vi "Offline_Analysis_SWSVM_newSelectionMethod_in_분석기.vi"(0 "LDA_matrix":path caption="LDA_matrix.txt", 1 "Target":path, 2 "Nontarget":path, 3 "in_matrix":path caption="in", 5 "svm_model_file":string, 7 "Target_order.txt":path, 9 "mius_flash_order":path, 11 "Brain":path, 12 "피험자이름":string="홍길동", 13 "Save_path":string) -> ()   [LabVIEW 2013]
uses:
  <vilib>/Utility/file.llb/Read From Spreadsheet File (DBL).vi
  <vilib>/Utility/file.llb/Read From Spreadsheet File (I64).vi
  <vilib>/Utility/file.llb/Write To Spreadsheet File (DBL).vi
  <vilib>/Utility/file.llb/Write To Spreadsheet File (I64).vi
  <vilib>/Utility/file.llb/Write To Spreadsheet File (string).vi
  <vilib>/Analysis/Matrix/NI_Matrix.lvlib
  <vilib>/Analysis/Matrix/Numeric/Conversions/Array To Matrix - RA2.vi
  <vilib>/Analysis/Matrix/Numeric/Conversions/Array To Matrix - RA.vi
panel:
  out "ACC":i16
  out "Target_order":i64[](array[numeric])
  out "Selected_Target":i32[](array[numeric])
  out "Accuracy":i16[](array[numeric])
  out "error out":errorcluster
  in  "Random_num":i32=6
  in  "Flash_Repeat":i32=20
  in  "Frame_Length":i32=10
  in  "Sampling_Rate":dbl=250.0
  # "ERP_Parameter안씀. LDA바로 집어넣으면 됨"
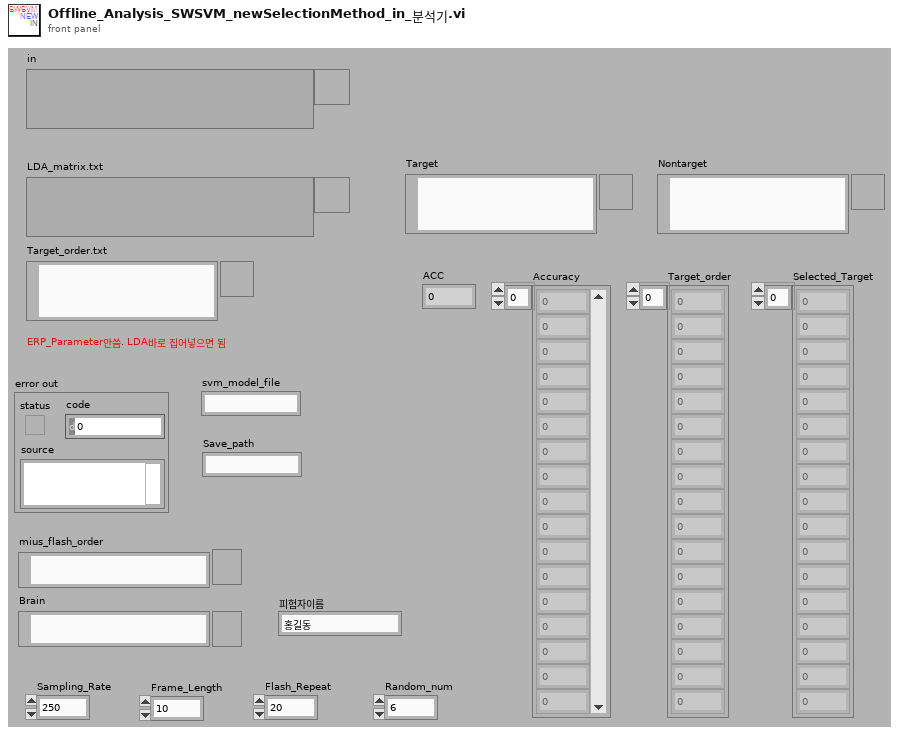
[diagram p1: front panel]
types:
  T1 = typedef "NI_Matrix.lvlib/RealMatrix.ctl" = dbl[][]
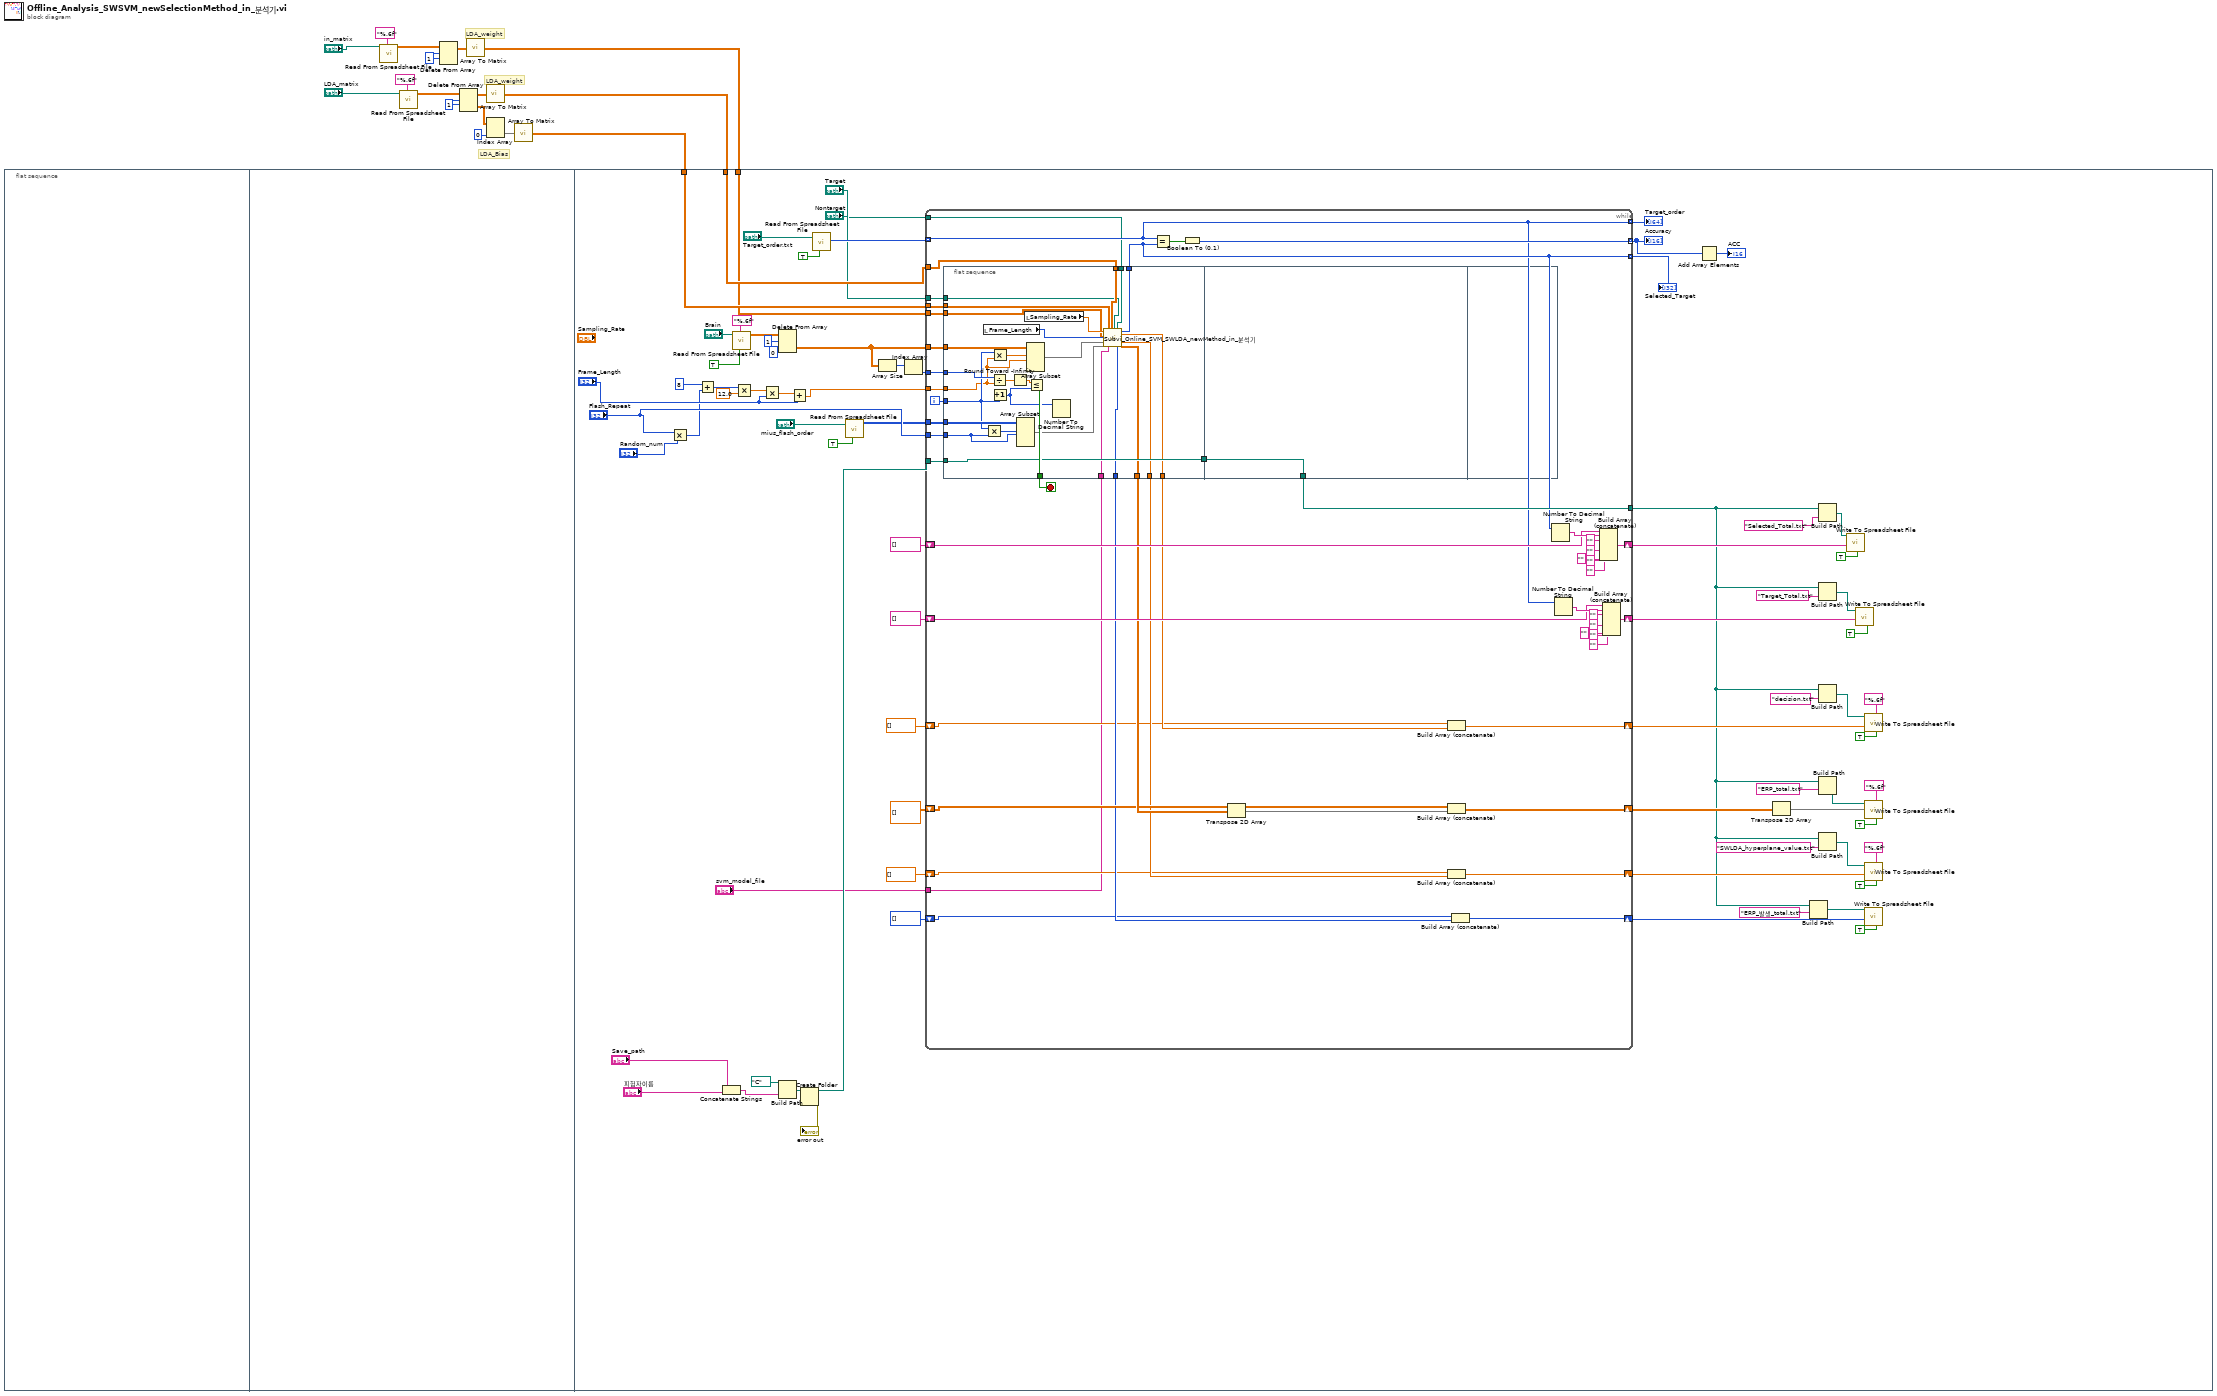
[diagram p0: block diagram]
diagram:
  w4 = 1 ("인덱스 (행)")
  w11 = 1 ("인덱스 (행)")
  # "LDA_weight"
  # "LDA_Bias"
  # "LDA_weight"
  n1 = flat-sequence {
    tunnel: w8 -> [w40]
    tunnel: w7 -> [w39]
    tunnel: w1 -> [w19]
    frame #0 {
    }
    frame #1 {
    }
    frame #2 {
      n2 = Multiply(x="Flash_Repeat", y="Random_num") -> (x*y=w80:i32)
      n3 = Add(x=8, y=w80) -> (x+y=w82:i32)
      n4 = Concatenate Strings("Save_path", "피험자이름") -> (w24:string)
      n5 = call-poly <vilib>:"Read From Spreadsheet File.vi"("transpose (no:F)"=TRUE, "format (%.3f)"="%.6f", "file path (dialog if empty)"="Brain") -> ("all rows"=w74:dbl[][])  [unwired: 4 in, 4 out]
      n6 = Multiply(x=w82, y=12.0) -> (x*y=w84:dbl)
      n7 = Multiply(x=w84, y="Frame_Length") -> (x*y=w86:dbl)
      n8 = Build Path(base path=path "C:/" ("path"), name or relative path=w24) -> (appended path=w89:path)
      n9 = Delete From Array(array=w74, length=1 ("길이"), index (col)=0 ("비활성화된 인덱스 (열)")) -> (deleted portion=w38:dbl[][])  [unwired: 1 in, 1 out]
      n10 = Add(x=w86, y="Frame_Length") -> (x+y=w87:dbl)
      n11 = Create Folder(path (use dialog)=w89) -> (created path=w91:path, error out=→"error out":errorcluster)  [unwired: 2 in, 1 out]
      n12 = call-poly <vilib>:"Read From Spreadsheet File.vi"("transpose (no:F)"=TRUE, "file path (dialog if empty)"="Target_order.txt") -> ("first row"=w68:i64[])  [unwired: 5 in, 4 out]
      n13 = call-poly <vilib>:"Read From Spreadsheet File.vi"("transpose (no:F)"=TRUE, "file path (dialog if empty)"="mius_flash_order") -> ("all rows"=w76:i64[][])  [unwired: 5 in, 4 out]
      n14 = Array Size(array=w38) -> (size(s)=w77:i32[])
      n15 = Index Array(array=w77) -> (element=w78:i32)  [unwired: 1 in]
      n16 = while {
        tunnel: w39 -> [w142]
        tunnel: w40 -> [w141]
        tunnel: w38 -> [w139]
        tunnel: w76 -> [w138]
        tunnel: w78 -> [w140]
        tunnel: w87 -> [w136]
        tunnel: "Flash_Repeat" -> [w137]
        tunnel: w91 -> [w135]
        tunnel: w68 -> [w113] mode=indexing
        tunnel: [w132] -> w60 mode=indexing
        tunnel: [w113] -> w65 mode=indexing
        tunnel: [w114] -> w66 mode=indexing
        tunnel: [w129] -> w26
        shift-right: [w116] -> w54
        shift-left: string[] [] -> [w115]
        shift-right: [w112] -> w53
        shift-left: string[] [] -> [w111]
        shift-right: [w108] -> w48
        shift-left: dbl[][] [] -> [w107]
        shift-right: [w105] -> w41
        shift-left: i16[] [] -> [w104]
        shift-right: [w102] -> w34
        shift-left: dbl[] [] -> [w101]
        shift-right: [w99] -> w27
        shift-left: dbl[] [] -> [w98]
        tunnel: "svm_model_file" -> [w97]
        tunnel: "Target" -> [w96]
        tunnel: "Nontarget" -> [w95]
        tunnel: w19 -> [w94]
        i -> [w131]
        stop <- w130 stop-if-true
        n17 = flat-sequence {
          tunnel: w142 -> [w170]
          tunnel: w141 -> [w169]
          tunnel: w140 -> [w168]
          tunnel: [w167] -> w130
          tunnel: w139 -> [w166]
          tunnel: w138 -> [w163]
          tunnel: w137 -> [w161]
          tunnel: w131 -> [w160]
          tunnel: w136 -> [w159]
          tunnel: w135 -> [w152]
          tunnel: [w152] -> w134
          tunnel: [w153] -> w114
          tunnel: [w151] -> w110
          tunnel: [w150] -> w106
          tunnel: [w148] -> w103
          tunnel: [w147] -> w100
          tunnel: w97 -> [w146]
          tunnel: w96 -> [w145]
          tunnel: w95 -> [w144]
          tunnel: w94 -> [w143]
          tunnel: w134 -> [w171]
          tunnel: [w171] -> w129
          frame #0 {
            n18 = local read "Frame_Length"() -> (w155:i32)
            n19 = Multiply(x=w160, y=w161) -> (x*y=w162:i32)
            n20 = Divide(x=w168, y=w159) -> (x/y=w158:dbl)
            n21 = Multiply(x=w160, y=w159) -> (x*y=w165:dbl)
            n22 = Increment(x=w160) -> (x+1=w154:i32)
            n23 = Round Toward -Infinity(1:w158) -> (0:w157:dbl)
            n24 = Array Subset(array=w163, index (row)=w162, length (row)=w161) -> (w149:i64[][])  [unwired: 2 in]
            n25 = local read "Sampling_Rate"() -> (w156:dbl)
            n26 = Array Subset(array=w166, index (row)=w165, length (row)=w159) -> (w164:dbl[][])  [unwired: 2 in]
            n27 = Less Or Equal?(x=w157, y=w154) -> (x <= y?=w167:bool)
            n28 = Number To Decimal String(number=w154) -> ()  [unwired: 1 in, 1 out]
            n29 = call "Subvi_Online_SVM_SWLDA_newMethod_in_분석기.vi"("rate"=w156, "samples per channel"=w155, "in"=w143, "Brain_data_source"=w164, "Target_Flash_Order"=w149, "Value"=w170, "svm_model_file"=w146, "Matrix"=w169, "Target"=w145, "Nontarget"=w144) -> ("EPR_발생_total"=w150:i16[], "output-0~8"=w153:i32, "decision"=w147:dbl[], "SWLDA"=w148:dbl[], "ERP_Parameters"=w151:dbl[][])  [unwired: 5 in]
          }
          frame #1 {
          }
          frame #2 {
          }
        }
        n30 = Equal?(x=w113, y=w114) -> (x = y?=w133:bool)
        n31 = Boolean To (0,1)(Boolean=w133) -> (0, 1=w132:i16)
        n32 = Transpose 2D Array(2D array=w110) -> (transposed array=w109:dbl[][])
        n33 = Build Array (concatenate)(w98, w100) -> (w99:dbl[])
        n34 = Build Array (concatenate)(w107, w109) -> (w108:dbl[][])
        n35 = Build Array (concatenate)(w101, w103) -> (w102:dbl[])
        n36 = Build Array (concatenate)(w104, w106) -> (w105:i16[])
        n37 = Number To Decimal String(number=w114) -> (decimal integer string=w122:string)  [unwired: 1 in]
        n38 = Number To Decimal String(number=w113) -> (decimal integer string=w128:string)  [unwired: 1 in]
        n39 = Build Array (concatenate)(w115, w122, "" ("element"), "" ("element"), "" ("element"), "" ("element"), "" ("element")) -> (w116:string[])
        n40 = Build Array (concatenate)(w111, w128, "" ("element"), "" ("element"), "" ("element"), "" ("element"), "" ("element")) -> (w112:string[])
      }
      "Accuracy" <- w60
      "Selected_Target" <- w66
      "Target_order" <- w65
      n41 = Add Array Elements(numeric array=w60) -> (sum=→"ACC":i16)
      n42 = Transpose 2D Array(2D array=w48) -> (transposed array=w46:dbl[][])
      n43 = Build Path(base path=w26, name or relative path="ERP_발생_total.txt") -> (appended path=w43:path)
      n44 = Build Path(base path=w26, name or relative path="Selected_Total.txt") -> (appended path=w56:path)
      n45 = Build Path(base path=w26, name or relative path="Target_Total.txt") -> (appended path=w62:path)
      n46 = Build Path(base path=w26, name or relative path="decision.txt") -> (appended path=w28:path)
      n47 = Build Path(base path=w26, name or relative path="ERP_total.txt") -> (appended path=w49:path)
      n48 = Build Path(base path=w26, name or relative path="SWLDA_hyperplane_value.txt") -> (appended path=w36:path)
      n49 = call-poly <vilib>:"Write To Spreadsheet File.vi"("transpose? (no:F)"=TRUE, "1D data"=w54, "file path (dialog if empty)"=w56) -> ()  [unwired: 5 in, 1 out]
      n50 = call-poly <vilib>:"Write To Spreadsheet File.vi"("transpose? (no:F)"=TRUE, "1D data"=w53, "file path (dialog if empty)"=w62) -> ()  [unwired: 5 in, 1 out]
      n51 = call-poly <vilib>:"Write To Spreadsheet File.vi"("transpose? (no:F)"=TRUE, "format (%.3f)"="%.6f", "1D data"=w27, "file path (dialog if empty)"=w28) -> ()  [unwired: 4 in, 1 out]
      n52 = call-poly <vilib>:"Write To Spreadsheet File.vi"("transpose? (no:F)"=TRUE, "format (%.3f)"="%.6f", "2D data"=w46, "file path (dialog if empty)"=w49) -> ()  [unwired: 4 in, 1 out]
      n53 = call-poly <vilib>:"Write To Spreadsheet File.vi"("transpose? (no:F)"=TRUE, "format (%.3f)"="%.6f", "1D data"=w34, "file path (dialog if empty)"=w36) -> ()  [unwired: 4 in, 1 out]
      n54 = call-poly <vilib>:"Write To Spreadsheet File.vi"("transpose? (no:F)"=TRUE, "1D data"=w41, "file path (dialog if empty)"=w43) -> ()  [unwired: 5 in, 1 out]
    }
  }
  n55 = call-poly <vilib>:"Read From Spreadsheet File.vi"("format (%.3f)"="%.6f", "file path (dialog if empty)"="in_matrix") -> ("all rows"=w3:dbl[][])  [unwired: 5 in, 4 out]
  n56 = call-poly <vilib>:"Read From Spreadsheet File.vi"("format (%.3f)"="%.6f", "file path (dialog if empty)"="LDA_matrix") -> ("all rows"=w9:dbl[][])  [unwired: 5 in, 4 out]
  n57 = Delete From Array(array=w3, length=w4, index (row)=w4) -> (array with subset deleted=w5:dbl[][])  [unwired: 1 in, 1 out]
  n58 = Delete From Array(array=w9, length=w11, index (row)=w11) -> (deleted portion=w14:dbl[][], array with subset deleted=w13:dbl[][])  [unwired: 1 in]
  n59 = call-poly <vilib>:"Array To Matrix.vi"("Real 2D Array"=w5) -> ("Real Matrix"=w1:T1)
  n60 = call-poly <vilib>:"Array To Matrix.vi"("Real 2D Array"=w13) -> ("Real Matrix"=w8:T1)
  n61 = Index Array(array=w14, index (col)=0 ("인덱스")) -> (element=w12:dbl[])  [unwired: 1 in]
  n62 = call-poly <vilib>:"Array To Matrix.vi"("Real 1D Array"=w12) -> ("Real Matrix (Column Vector)"=w7:T1)
